vi "connectCommandSubscribe.vi"(8 "error in (no error)":errorcluster, 11 "MiddlewareSVThisComponent in":refnum<class "MiddlewareSVThisComponent.lvclass">) -> (0 "error out":errorcluster, 3 "MiddlewareSVThisComponent out":refnum<class "MiddlewareSVThisComponent.lvclass">)   [LabVIEW 2015, in "MiddlewareSVThisComponent.lvclass"]
uses:
  MiddlewareSVThisComponent.lvclass
  ComponentTemplateCore/ComponentModel/ComponentModel/Typedefs/HeartbeatConfig.ctl
  ComponentTemplateCore/ComponentModel/ComponentModel/Typedefs/SVProcessConfig.ctl
  ComponentTemplateCore/ComponentModel/ComponentModel/Typedefs/CommunicationConfig.ctl
  ComponentTemplateCore/ComponentModel/ComponentModel/MiddlewareSV/MiddlewareSV.lvclass/MiddlewareSV.ctl
  ComponentTemplateCore/ComponentModel/ComponentModel/Middleware/Middleware.lvclass/Middleware.ctl
  ComponentTemplateCore/ComponentModel/ComponentModel/InternalSignals/clearMessagingError.vi
  ComponentTemplateCore/ComponentModel/ComponentModel/MiddlewareSV/MiddlewareSV.lvclass
  ComponentTemplateCore/ComponentModel/ComponentModel/InternalSignals/InternalSignalsGlobals.lvlib
  ComponentTemplateCore/ComponentModel/ComponentModelDT/ConfigurationFileReaderDT/ConfigurationFileReaderDT.lvclass
  ComponentTemplateCore/ComponentModel/ComponentModel/Middleware/Middleware.lvclass
  ComponentTemplateCore/ComponentModel/ComponentModelRT/ConfigurationFileReaderRT/ConfigurationFileReaderRT.lvclass
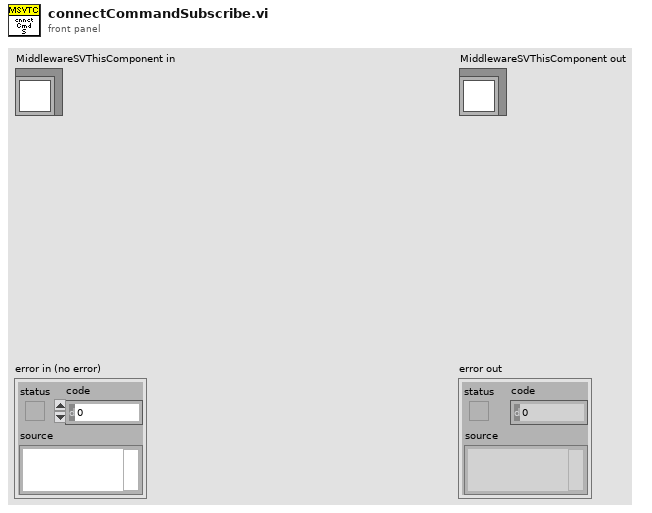
[diagram p1: front panel]
types:
  T1 = typedef "CommunicationConfig.ctl" = cluster{"hostComputerAddress":string, "ComponentAcronym":string, "InstanceIdentifier":i32}
  T2 = typedef "SVProcessConfig.ctl" = cluster{"subDataProcessPrototype":string, "pubDataProcessPrototype":string, "commandProcessPrototype":string, "commandSVName":string}
  T3 = typedef "heartbeatConfig.ctl" = cluster{"Heartbeat Interval (s)":dbl, "Heartbeat Timeout (s)":dbl}
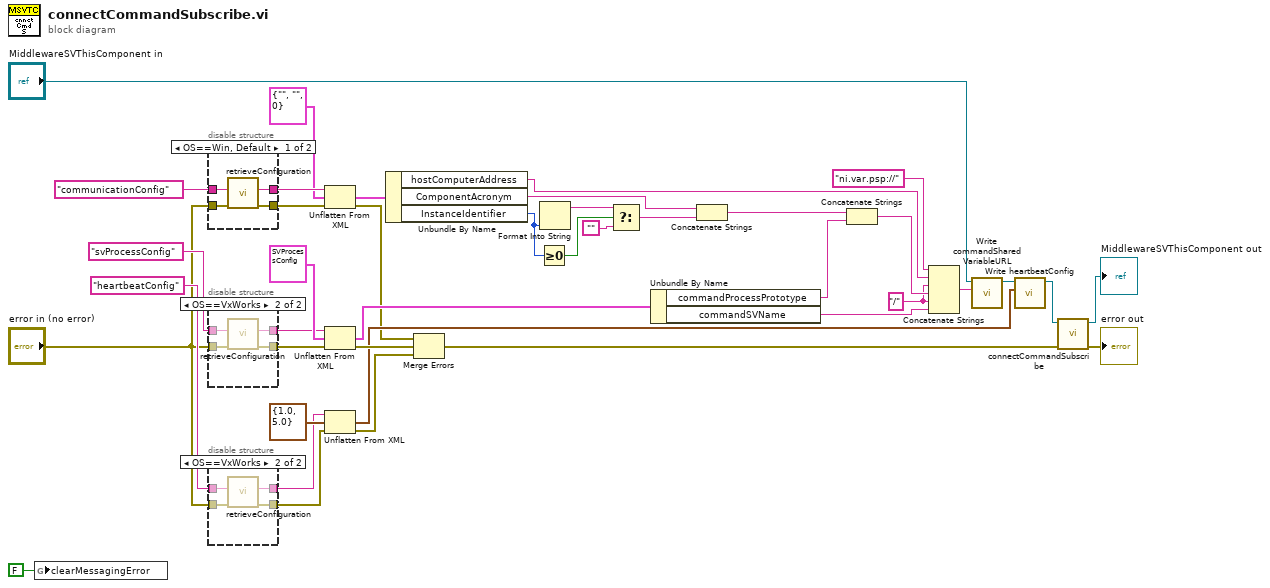
[diagram p0: block diagram]
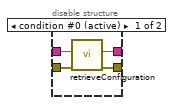
[diagram p2: hidden frame]
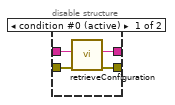
[diagram p3: hidden frame]
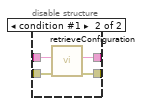
[diagram p4: hidden frame]
diagram:
  w35 = "/" ("string")
  n1 = global write "clearMessagingError.vi" "clearMessagingError"(FALSE ("clearMessagingError")) -> ()
  n2 = disable-structure shown="OS==Win, Default" {
    disable-tunnel: "communicationConfig" ("dataName") -> [w44 w48]
    disable-tunnel: [w43 w46] -> w26
    disable-tunnel: [w42 w45] -> w23
    disable-tunnel: "error in (no error)" -> [w41 w47]
    frame condition #0 (active) {
      n3 = call "retrieveConfiguration.vi"("error in (no error)"=w41, "dataName"=w44) -> ("error out"=w42:errorcluster, "dataValueFromFile"=w43:string)  [unwired: 7 in, 1 out]
    }
    frame condition #1 {
      n4 = call "retrieveConfiguration.vi"("error in (no error)"=w47, "dataName"=w48) -> ("error out"=w45:errorcluster, "dataValueFromFile"=w46:string)  [unwired: 7 in, 1 out]
    }
  }
  n5 = disable-structure shown="OS==VxWorks" {
    disable-tunnel: "svProcessConfig" ("dataName") -> [w52 w56]
    disable-tunnel: [w51 w54] -> w6
    disable-tunnel: [w50 w53] -> w8
    disable-tunnel: "error in (no error)" -> [w49 w55]
    frame condition #0 (active) {
      n6 = call "retrieveConfiguration.vi"("error in (no error)"=w49, "dataName"=w52) -> ("error out"=w50:errorcluster, "dataValueFromFile"=w51:string)  [unwired: 7 in, 1 out]
    }
    frame condition #1 {
      n7 = call "retrieveConfiguration.vi"("error in (no error)"=w55, "dataName"=w56) -> ("error out"=w53:errorcluster, "dataValueFromFile"=w54:string)  [unwired: 7 in, 1 out]
    }
  }
  n8 = disable-structure shown="OS==VxWorks" {
    disable-tunnel: "heartbeatConfig" ("dataName") -> [w60 w64]
    disable-tunnel: [w59 w62] -> w3
    disable-tunnel: [w58 w61] -> w4
    disable-tunnel: "error in (no error)" -> [w57 w63]
    frame condition #0 (active) {
      n9 = call "retrieveConfiguration.vi"("error in (no error)"=w57, "dataName"=w60) -> ("error out"=w58:errorcluster, "dataValueFromFile"=w59:string)  [unwired: 7 in, 1 out]
    }
    frame condition #1 {
      n10 = call "retrieveConfiguration.vi"("error in (no error)"=w63, "dataName"=w64) -> ("error out"=w61:errorcluster, "dataValueFromFile"=w62:string)  [unwired: 7 in, 1 out]
    }
  }
  n11 = Unflatten From XML(xml string=w26, type=T1 {"hostComputerAddress"="", "ComponentAcronym"="", "InstanceIdentifier"=0} ("communicationConfig"), error in (no error)=w23) -> (value=w34:T1, error out=w1:errorcluster)
  n12 = Unflatten From XML(xml string=w6, type=T2 {"subDataProcessPrototype"="SubDataSV", "pubDataProcessPrototype"="PubDataSV", "commandProcessPrototype"="CommandSV", "commandSVName"="Command"} ("svProcessConfig"), error in (no error)=w8) -> (value=w21:T2, error out=w18:errorcluster)
  n13 = Unflatten From XML(xml string=w3, type=T3 {"Heartbeat Interval (s)"=1.0, "Heartbeat Timeout (s)"=5.0} ("heartbeatConfig"), error in (no error)=w4) -> (value=w10:T3, error out=w24:errorcluster)
  n14 = Unbundle By Name(w34) -> ("hostComputerAddress"=w36:string, "ComponentAcronym"=w37:string, "InstanceIdentifier"=w33:i32)
  n15 = Merge Errors(w1, w18, w24) -> (w13:errorcluster)
  n16 = Greater Or Equal To 0?(x=w33) -> (x >= 0?=w31:bool)
  n17 = Format Into String(w33) -> (resulting string=w32:string)  [unwired: 3 in, 1 out]
  n18 = Select(t=w32, s=w31, f="") -> (s? t:f=w29:string)
  n19 = Unbundle By Name(w21) -> ("commandProcessPrototype"=w20:string, "commandSVName"=w19:string)
  n20 = Concatenate Strings(w37, w29) -> (w39:string)
  n21 = Concatenate Strings(w39, w20) -> (w40:string)
  n22 = Concatenate Strings("ni.var.psp://" ("string"), w36, w35, w40, w35, w19) -> (w15:string)
  n23 = call "Write commandSharedVariableURL.vi"("commandSharedVariableURL"=w15, "MiddlewareSV in"="MiddlewareSVThisComponent in") -> ("MiddlewareSV out"=w11:refnum<class "MiddlewareSVThisComponent.lvclass">)  [unwired: 9 in]
  n24 = call "Write heartbeatConfig.vi"("heartbeatConfig"=w10, "Middleware in"=w11) -> ("Middleware out"=w9:refnum<class "MiddlewareSVThisComponent.lvclass">)  [unwired: 9 in]
  n25 = call-parent "connectCommandSubscribe.vi"("error in (no error)"=w13, "MiddlewareSV in"=w9) -> ("error out"=→"error out":errorcluster, "MiddlewareSV out"=→"MiddlewareSVThisComponent out":refnum<class "MiddlewareSVThisComponent.lvclass">)  [unwired: 8 in]
